vi "Main.vi"() -> ()   [LabVIEW 2016]
uses:
  Experiment States.ctl
  <vilib>/DAQmx/write.llb/DAQmx Write (Analog 1D DBL NChan 1Samp).vi
  <vilib>/DAQmx/read.llb/DAQmx Read (Analog 2D DBL NChan NSamp).vi
  <vilib>/DAQmx/read.llb/DAQmx Read (Analog 1D DBL 1Chan NSamp).vi
  <vilib>/DAQmx/miscellaneous.llb/DAQmx Fill In Error Info.vi
panel:
  in  "Mass Flow Controller 1 Output Channel":tag
  in  "Mass Flow Controller 2 Output Channel":tag
  in  "Mass Flow Controller 2 Setpoint":dbl
  in  "Mass Flow Controller 1 Setpoint":dbl
  out "Mass Flow Controller 2":dbl(knob) scale=0.0..500.0
  out "Mass Flow Controller 1":dbl(knob) scale=0.0..200.0
  in  "Mass Flow Controller 2 Input Channel":tag
  in  "Mass Flow Controller 1 Input Channel":tag
  in  "Thermocouple 1 Channel":tag
  out "Waveform Chart":dbl(graph)
  out "Thermocouple":dbl(slide) scale=0.0..100.0
  in  "Skip Export":bool
  in  "End Experiment?":bool
  in  "Export?":bool
  in  "Start":bool
  # "Set all of the above values before starting the experiment!"
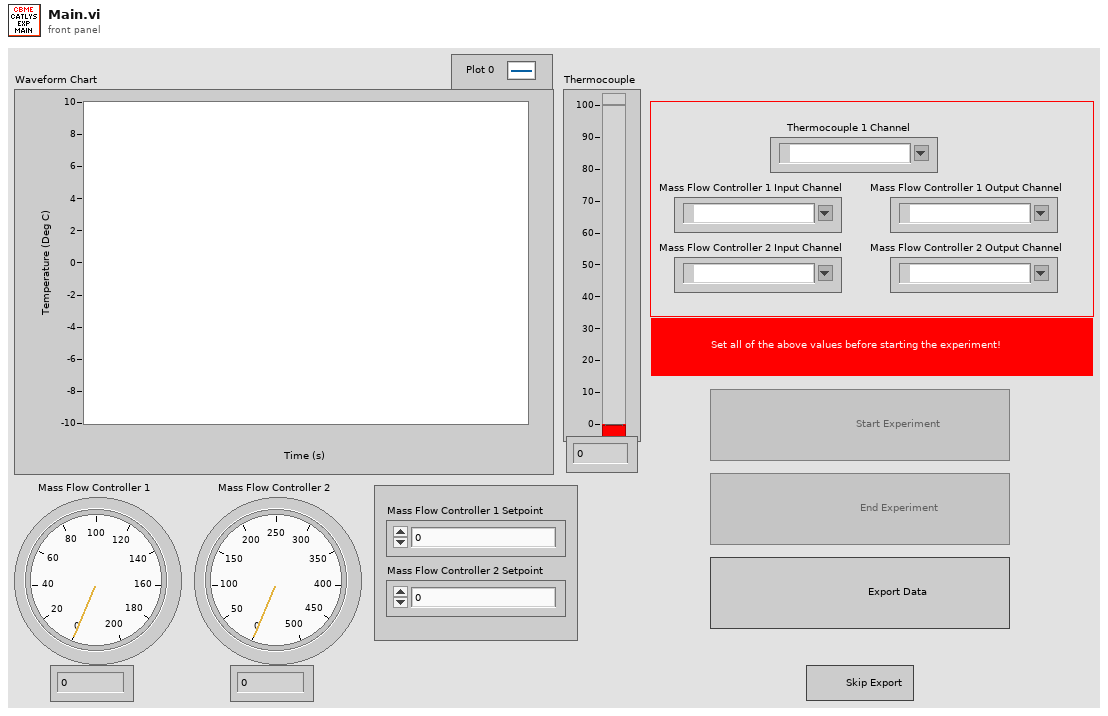
[diagram p1: front panel]
types:
  T1 = typedef "Experiment States.ctl" = enum16{"Setup", "Data Collection", "Export", "Finish"}
  T2 = enum8{"Enabled", "Disabled", "Disabled and Grayed Out"}
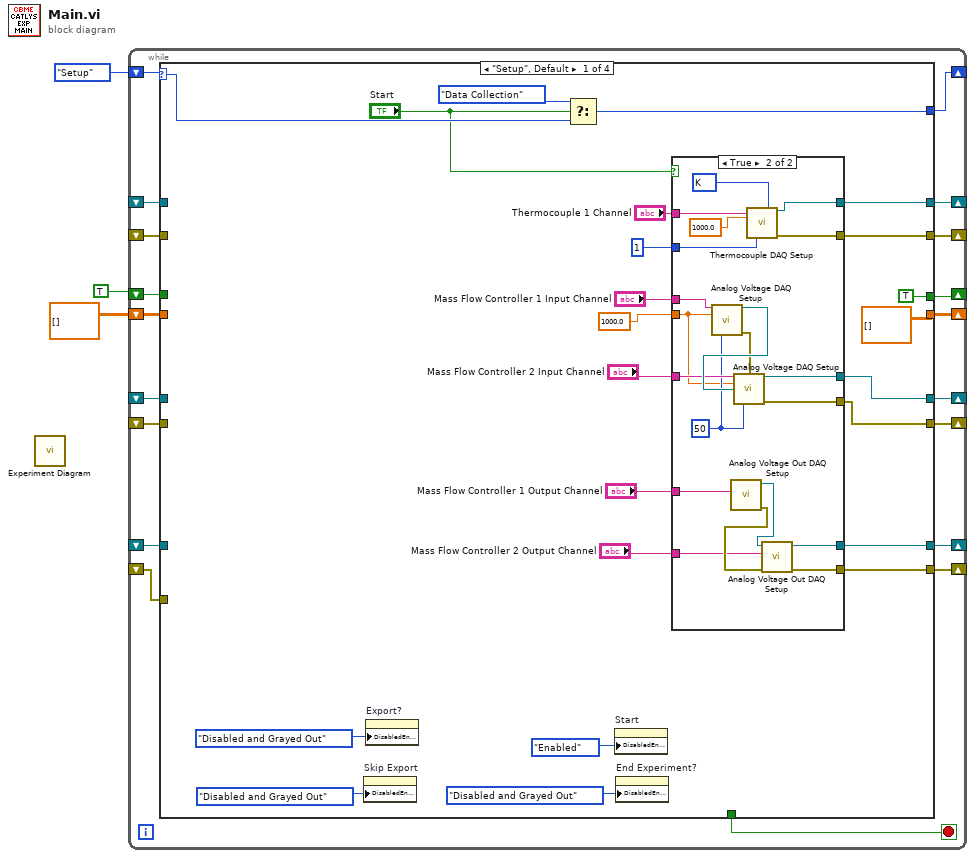
[diagram p0: block diagram]
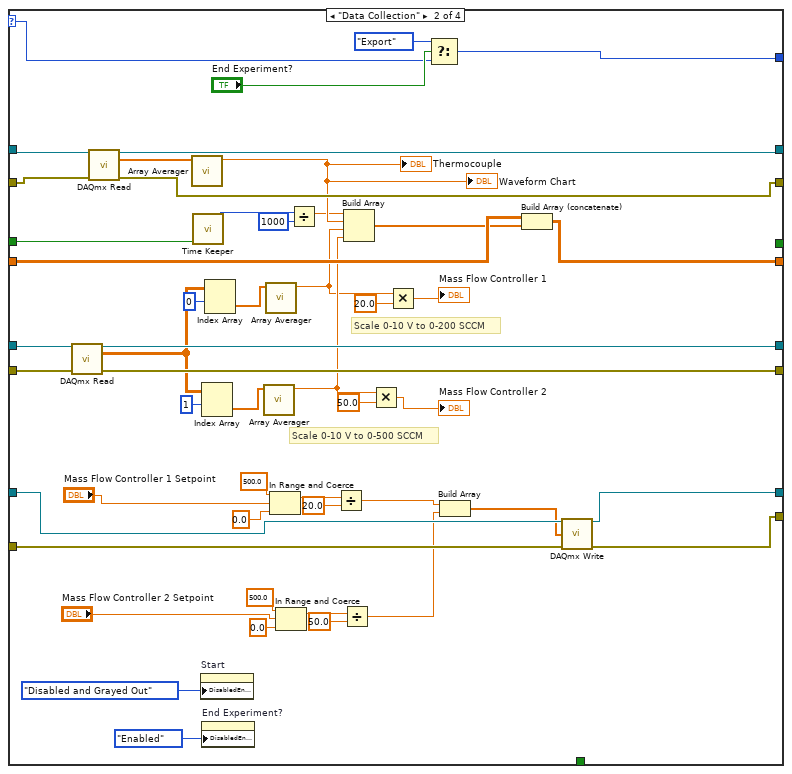
[diagram p3: hidden frame]
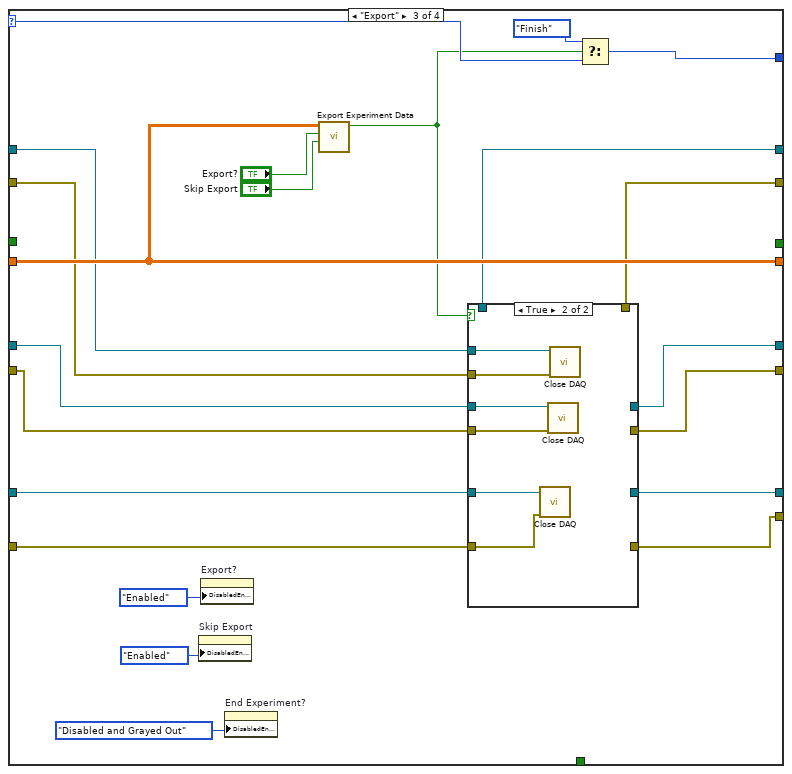
[diagram p4: hidden frame]
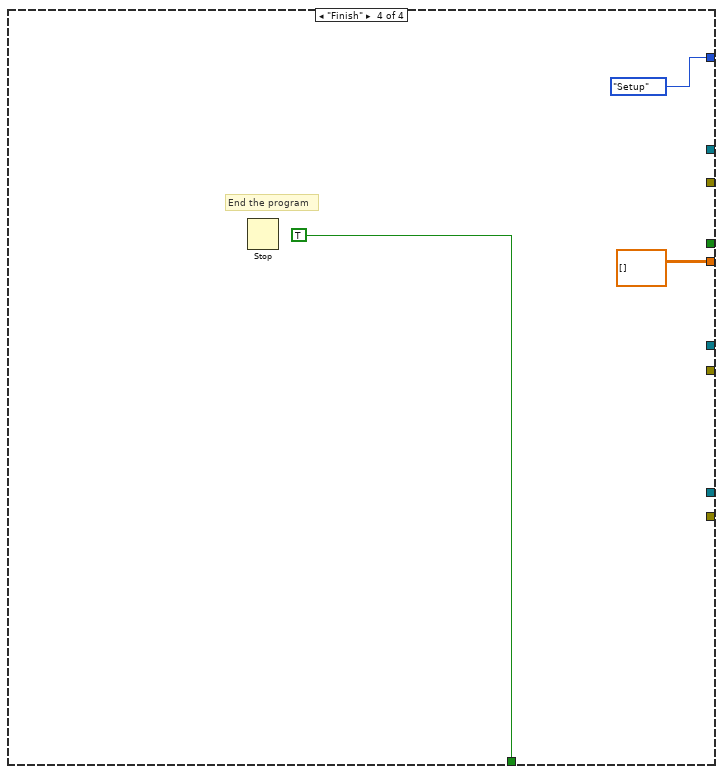
[diagram p6: hidden frame]
diagram:
  n1 = call "Experiment Diagram.vi"() -> ()  [unwired: 12 in]
  n2 = while {
    shift-right: [w21] -> _
    shift-left: Experiment_States."Setup" ("Enum") -> [w22]
    shift-right: [w19] -> _
    shift-left: _ -> [w17]
    shift-right: [w18] -> _
    shift-left: _ -> [w16]
    shift-right: [w12] -> _
    shift-left: dbl[][] [] -> [w13]
    shift-right: [w14] -> _
    shift-left: TRUE -> [w15]
    shift-right: [w11] -> _
    shift-left: _ -> [w9]
    shift-right: [w10] -> _
    shift-left: _ -> [w8]
    shift-right: [w7] -> _
    shift-left: _ -> [w5]
    shift-right: [w6] -> _
    shift-left: _ -> [w4]
    stop <- w20 stop-if-true
    n3 = case shown="\"Setup\", Default" w22 {
      selector: w22 -> [w45 w115 w136 _]
      tunnel: [w43 w113 w134 Experiment_States."Setup" ("Enum")] -> w21
      tunnel: [_ _ _ TRUE] -> w20
      tunnel: [w38 w107 w125 _] -> w19
      tunnel: [w35 w106 w124 _] -> w18
      tunnel: w17 -> [_ w110 w131 _]
      tunnel: w16 -> [_ w109 w130 _]
      tunnel: w15 -> [_ w105 _ _]
      tunnel: [TRUE _ _ _] -> w14
      tunnel: w13 -> [_ w100 w133 _]
      tunnel: [dbl[][] [] w98 w133 dbl[][] []] -> w12
      tunnel: [w28 w95 w123 _] -> w11
      tunnel: [w27 w94 w122 _] -> w10
      tunnel: w9 -> [_ w97 w129 _]
      tunnel: w8 -> [_ w96 w128 _]
      tunnel: [w24 w70 w121 _] -> w7
      tunnel: [w23 w69 w120 _] -> w6
      tunnel: w5 -> [_ w72 w127 _]
      tunnel: w4 -> [_ w71 w126 _]
      frame "Setup", Default {
        n4 = property on="Skip Export" class="Bool"("DisabledEnum"=T2."Disabled and Grayed Out" ("Disabled")) -> ()  [unwired: 2 in, 2 out]
        n5 = property on="Export?" class="Bool"("DisabledEnum"=T2."Disabled and Grayed Out" ("Disabled")) -> ()  [unwired: 2 in, 2 out]
        n6 = Select(t=Experiment_States."Data Collection", s="Start", f=w45) -> (s? t:f=w43:T1)
        n7 = property on="Start" class="Bool"("DisabledEnum"=T2."Enabled" ("Disabled")) -> ()  [unwired: 2 in, 2 out]
        n8 = property on="End Experiment?" class="Bool"("DisabledEnum"=T2."Disabled and Grayed Out" ("Disabled")) -> ()  [unwired: 2 in, 2 out]
        n9 = case shown="True" "Start" {
          tunnel: [_ w65] -> w38
          tunnel: "Thermocouple 1 Channel" -> [_ w64]
          tunnel: 1 ("samples per channel") -> [_ w62]
          tunnel: [_ w61] -> w35
          tunnel: "Mass Flow Controller 1 Input Channel" -> [_ w57]
          tunnel: "Mass Flow Controller 2 Input Channel" -> [_ w56]
          tunnel: 1000.0 ("Sample Rate") -> [_ w54]
          tunnel: [_ w53] -> w28
          tunnel: [_ w52] -> w27
          tunnel: "Mass Flow Controller 1 Output Channel" -> [_ w51]
          tunnel: "Mass Flow Controller 2 Output Channel" -> [_ w48]
          tunnel: [_ w47] -> w24
          tunnel: [_ w46] -> w23
          frame False {
          }
          frame True {
            w55 = 50 ("samples per channel")
            w63 = 10073 items=["J"=10072, "K"=10073, "N"=10077, "R"=10082, "S"=10085, "T"=10086, "B"=10047, "E"=10055] ("Thermocouple Type")
            n10 = call "Analog Voltage DAQ Setup.vi"("physical channels"=w57, "Sample Rate"=w54, "samples per channel"=w55) -> ("task out"=w59:refnum<k21>, "error out"=w58:errorcluster)  [unwired: 11 in]
            n11 = call "Analog Voltage Out DAQ Setup.vi"("physical channels"=w51) -> ("error out"=w50:errorcluster, "task out"=w49:refnum<k21>)  [unwired: 9 in]
            n12 = call "Analog Voltage DAQ Setup.vi"("physical channels"=w56, "error in"=w58, "Sample Rate"=w54, "task in"=w59, "samples per channel"=w55) -> ("task out"=w53:refnum<k21>, "error out"=w52:errorcluster)  [unwired: 9 in]
            n13 = call "Thermocouple DAQ Setup.vi"("physical channels"=w64, "Thermocouple Type"=w63, "Sample Rate"=1000.0, "samples per channel"=w62) -> ("task out"=w65:refnum<k21>, "error out"=w61:errorcluster)  [unwired: 10 in]
            n14 = call "Analog Voltage Out DAQ Setup.vi"("error in"=w50, "physical channels"=w48, "task in"=w49) -> ("error out"=w46:errorcluster, "task out"=w47:refnum<k21>)  [unwired: 7 in]
          }
        }
      }
      frame "Data Collection" {
        # "Scale 0-10 V to 0-200 SCCM"
        # "Scale 0-10 V to 0-500 SCCM"
        n15 = call-poly <vilib>:"DAQmx Read.vi"("task/channels in"=w97, "error in"=w96) -> ("task out"=w95:refnum<k21>, "data"=w93:dbl[][], "error out"=w94:errorcluster)  [unwired: 11 in]
        n16 = call-poly <vilib>:"DAQmx Read.vi"("task/channels in"=w110, "error in"=w109) -> ("task out"=w107:refnum<k21>, "data"=w108:dbl[], "error out"=w106:errorcluster)  [unwired: 11 in]
        n17 = call "Array Averager.vi"("Array"=w108) -> ("Averaged Array"=w104:dbl)  [unwired: 10 in]
        "Thermocouple" <- w104
        "Waveform Chart" <- w104
        n18 = call "Time Keeper.vi"("Reset?"=w105) -> ("Time Elapsed (ms)"=w103:u32)  [unwired: 10 in]
        n19 = property on="Start" class="Bool"("DisabledEnum"=T2."Disabled and Grayed Out" ("Disabled")) -> ()  [unwired: 2 in, 2 out]
        n20 = Index Array(array=w93, index (row)=1) -> (element=w90:dbl[])  [unwired: 1 in]
        n21 = property on="End Experiment?" class="Bool"("DisabledEnum"=T2."Enabled" ("Disabled")) -> ()  [unwired: 2 in, 2 out]
        n22 = Index Array(array=w93, index (row)=0) -> (element=w89:dbl[])  [unwired: 1 in]
        n23 = call "Array Averager.vi"("Array"=w90) -> ("Averaged Array"=w88:dbl)  [unwired: 10 in]
        n24 = call "Array Averager.vi"("Array"=w89) -> ("Averaged Array"=w83:dbl)  [unwired: 10 in]
        n25 = In Range and Coerce(upper limit=500.0, x="Mass Flow Controller 1 Setpoint", lower limit=0.0) -> (coerced(x)=w76:dbl)  [unwired: 1 out]
        n26 = In Range and Coerce(upper limit=500.0, x="Mass Flow Controller 2 Setpoint", lower limit=0.0) -> (coerced(x)=w79:dbl)  [unwired: 1 out]
        n27 = Divide(x=w103, y=u32 1000) -> (x/y=w101:dbl)
        n28 = Divide(x=w76, y=20.0) -> (x/y=w68:dbl)
        n29 = Divide(x=w79, y=50.0) -> (x/y=w67:dbl)
        n30 = Build Array(w101, w104, w83, w88) -> (w99:dbl[])
        n31 = Multiply(x=w88, y=50.0) -> (x*y=→"Mass Flow Controller 2":dbl)
        n32 = Multiply(x=w83, y=20.0) -> (x*y=→"Mass Flow Controller 1":dbl)
        n33 = Select(t=Experiment_States."Export", s="End Experiment?", f=w115) -> (s? t:f=w113:T1)
        n34 = Build Array(w68, w67) -> (w66:dbl[])
        n35 = Build Array (concatenate)(w100, w99) -> (w98:dbl[][])
        n36 = call-poly <vilib>:"DAQmx Write.vi"("task/channels in"=w72, "data"=w66, "error in"=w71) -> ("task out"=w70:refnum<k21>, "error out"=w69:errorcluster)  [unwired: 10 in, 1 out]
      }
      frame "Export" {
        n37 = property on="Skip Export" class="Bool"("DisabledEnum"=T2."Enabled" ("Disabled")) -> ()  [unwired: 2 in, 2 out]
        n38 = property on="Export?" class="Bool"("DisabledEnum"=T2."Enabled" ("Disabled")) -> ()  [unwired: 2 in, 2 out]
        n39 = property on="End Experiment?" class="Bool"("DisabledEnum"=T2."Disabled and Grayed Out" ("Disabled")) -> ()  [unwired: 2 in, 2 out]
        n40 = call "Export Experiment Data.vi"("Skip Export"="Skip Export", "Export?"="Export?", "Data"=w133) -> ("Export Complete?"=w132:bool)  [unwired: 8 in]
        n41 = case shown="True" w132 {
          tunnel: w131 -> [w144 w150]
          tunnel: w130 -> [w143 w149]
          tunnel: w129 -> [w142 w148]
          tunnel: w128 -> [w141 w147]
          tunnel: w127 -> [w140 w146]
          tunnel: w126 -> [w139 w145]
          tunnel: [w144 _] -> w125
          tunnel: [w143 _] -> w124
          tunnel: [w142 _] -> w123
          tunnel: [w141 _] -> w122
          tunnel: [w140 _] -> w121
          tunnel: [w139 _] -> w120
          frame False {
          }
          frame True {
            n42 = call "Close DAQ.vi"("error in (no error)"=w145, "Refnum in"=w146) -> ()  [unwired: 10 in]
            n43 = call "Close DAQ.vi"("error in (no error)"=w147, "Refnum in"=w148) -> ()  [unwired: 10 in]
            n44 = call "Close DAQ.vi"("error in (no error)"=w149, "Refnum in"=w150) -> ()  [unwired: 10 in]
          }
        }
        n45 = Select(t=Experiment_States."Finish", s=w132, f=w136) -> (s? t:f=w134:T1)
      }
      frame "Finish" {
        # "End the program"
        n46 = Stop() -> ()  [unwired: 1 in]
      }
    }
  }
